vi "Edit Frame.vi"(8 "error in (no error)":errorcluster, 11 "Node Ptr":u64 format="%.0x") -> (0 "error out":errorcluster)   [LabVIEW 2015, in "Diagnostics Addon System Explorer.lvlib"]
uses:
  Diagnostics Addon System Explorer.lvlib
  Types/FG.Action.ctl
  SubVIs/Signal.FG.vi
  Shared/SubVIs/Constants.vi
  <vilib>/NI Veristand/Custom Device API/NI VeriStand - Set Item Property.vi
  <vilib>/NI Veristand/Custom Device API/Set Item Property (U32).vi
  <vilib>/NI Veristand/Custom Device API/Set Item Property (Double).vi
  <vilib>/NI Veristand/Custom Device API/Set Item Property (String).vi
  <vilib>/NI Veristand/Custom Device API/NI VeriStand - Get Item Property.vi
  <vilib>/NI Veristand/Custom Device API/Get Item Property (U32).vi
  <vilib>/NI Veristand/Custom Device API/Get Item Property (Double).vi
  <vilib>/NI Veristand/Custom Device API/Get Item Property (String).vi
  <vilib>/NI Veristand/Custom Device API/NI VeriStand - Get Item Description.vi
  <vilib>/NI Veristand/Custom Device API/NI VeriStand - Get Custom Device Channel Data.vi
  <vilib>/NI Veristand/Custom Device API/Custom Device API.lvlib
  Shared/Diagnostics Addon Shared.lvlib
  <vilib>/NI Veristand/Custom Device Tools/Custom Device Utility Library/Custom Device Utility Library.lvlib
panel:
  in  "Tag":string
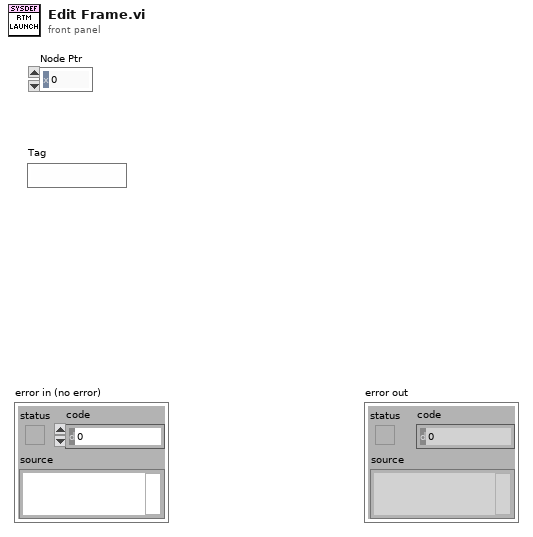
[diagram p1: front panel]
types:
  T1 = typedef "Diagnostics Addon Shared.lvlib/Signal.ctl" = cluster{"Start Bit":u32, "Length":u32, "Scaling Factor":dbl, "Scaling Offset":dbl, "Minimum":dbl, "Maximum":dbl, "Data Type":u32, "Byte Order":u32, "Default Value":dbl, "Name":string, "Units":string, "Description":string}
  T2 = typedef "Custom Device API.lvlib/Custom Device Item Ref.ctl" = u64
  T3 = typedef "Custom Device API.lvlib/Custom Device Item Info.ctl" = cluster{"Name":string, "Is Channel":bool, "GUID":string, "Is Waveform":bool}
  T4 = typedef "Diagnostics Addon System Explorer.lvlib/FG.Action.ctl" = enum16{"Get", "Set"}
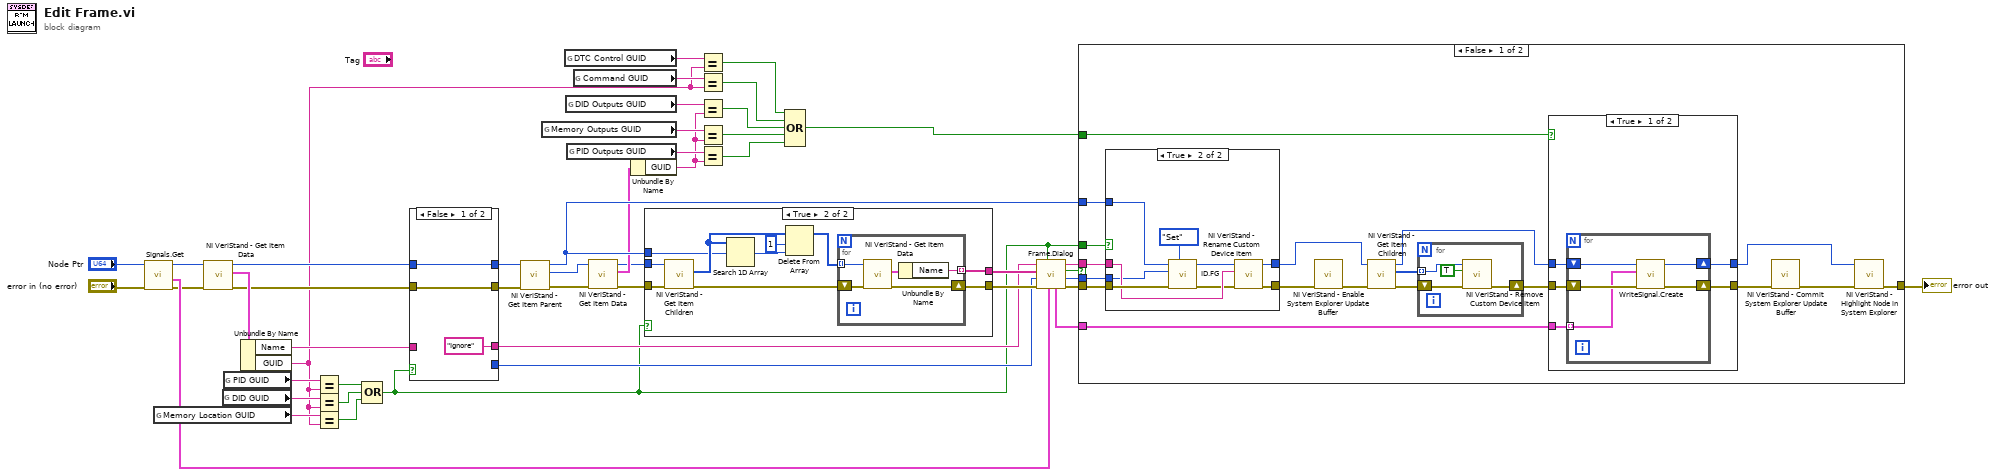
[diagram p0: block diagram]
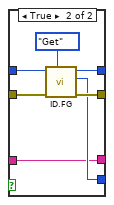
[diagram p3: hidden frame]
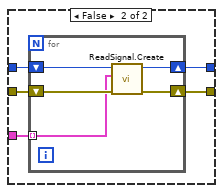
[diagram p5: hidden frame]
diagram:
  n1 = call "Signals.Get.vi"("error in (no error)"="error in (no error)", "Device Item Ref out"="Node Ptr") -> ("error out"=w28:errorcluster, "Parameters"=w30:T1[], "Item Ref out"=w29:T2)  [unwired: 6 in, 1 out]
  n2 = global read "Constants.vi" "Memory Location GUID"() -> (w9:string)
  n3 = call <vilib>:"NI VeriStand - Get Item Data.vi"("error in (no error)"=w28, "Item Ref in"=w29) -> ("error out"=w23:errorcluster, "Item Info"=w26:T3, "Item Ref out"=w24:T2)  [unwired: 6 in, 1 out]
  n4 = global read "Constants.vi" "DID GUID"() -> (w27:string)
  n5 = global read "Constants.vi" "PID GUID"() -> (w25:string)
  n6 = Unbundle By Name(w26) -> ("Name"=w17:string, "GUID"=w4:string)
  n7 = Equal?(x=w25, y=w4) -> (x = y?=w22:bool)
  n8 = Equal?(x=w27, y=w4) -> (x = y?=w21:bool)
  n9 = Equal?(x=w9, y=w4) -> (x = y?=w8:bool)
  n10 = Compound Arithmetic op=OR(w22, w21, w8) -> (w12:bool)
  n11 = case shown="False" w12 {
    tunnel: w24 -> [w49 w52]
    tunnel: w23 -> [w50 w53]
    tunnel: [w50 w56] -> w20
    tunnel: [w49 w55] -> w19
    tunnel: [_ w54] -> w18
    tunnel: ["Ignore" ("Name") w51] -> w16
    tunnel: w17 -> [_ w51]
    frame False {
    }
    frame True {
      n12 = call "ID.FG.vi"("Action"=FG.Action."Get", "error in (no error)"=w53, "Device Item Ref in"=w52) -> ("error out"=w56:errorcluster, "ID"=w54:u32, "Device Item Ref out"=w55:T2)  [unwired: 6 in]
    }
  }
  n13 = call <vilib>:"NI VeriStand - Get Item Parent.vi"("error in (no error)"=w20, "Item Ref in"=w19) -> ("error out"=w38:errorcluster, "Parent Ref"=w37:T2, "Item Ref out"=w42:T2)  [unwired: 6 in, 1 out]
  n14 = global read "Constants.vi" "Memory Outputs GUID"() -> (w10:string)
  n15 = global read "Constants.vi" "DTC Control GUID"() -> (w5:string)
  n16 = global read "Constants.vi" "DID Outputs GUID"() -> (w7:string)
  n17 = global read "Constants.vi" "PID Outputs GUID"() -> (w39:string)
  n18 = global read "Constants.vi" "Command GUID"() -> (w15:string)
  n19 = call <vilib>:"NI VeriStand - Get Item Data.vi"("error in (no error)"=w38, "Item Ref in"=w37) -> ("error out"=w35:errorcluster, "Item Info"=w40:T3, "Item Ref out"=w36:T2)  [unwired: 6 in, 1 out]
  n20 = Unbundle By Name(w40) -> ("GUID"=w6:string)
  n21 = case shown="True" w12 {
    tunnel: [w58 w63] -> w44
    tunnel: [_ w62] -> w43
    tunnel: w42 -> [_ w61]
    tunnel: w36 -> [_ w60]
    tunnel: w35 -> [w58 w59]
    frame False {
    }
    frame True {
      n22 = call <vilib>:"NI VeriStand - Get Item Children.vi"("error in (no error)"=w59, "Item Ref in"=w60) -> ("error out"=w68:errorcluster, "Child Refs"=w67:T2[])  [unwired: 6 in, 2 out]
      n23 = Search 1D Array(1D array=w67, element=w61) -> (index of element=w65:i32)  [unwired: 1 in]
      n24 = Delete From Array(array=w67, length=1, index=w65) -> (array with subset deleted=w66:T2[])  [unwired: 1 out]
      n25 = for {
        tunnel: [w71] -> w62 mode=indexing
        shift-right: [w70] -> w63
        shift-left: w68 -> [w72]
        tunnel: w66 -> [w69] mode=indexing
        n26 = call <vilib>:"NI VeriStand - Get Item Data.vi"("error in (no error)"=w72, "Item Ref in"=w69) -> ("error out"=w70:errorcluster, "Item Info"=w73:T3)  [unwired: 8 out]
        n27 = Unbundle By Name(w73) -> ("Name"=w71:string)
      }
    }
  }
  n28 = Equal?(x=w5, y=w4) -> (x = y?=w1:bool)
  n29 = Equal?(x=w15, y=w4) -> (x = y?=w3:bool)
  n30 = Equal?(x=w7, y=w6) -> (x = y?=w2:bool)
  n31 = Equal?(x=w10, y=w6) -> (x = y?=w11:bool)
  n32 = Equal?(x=w39, y=w6) -> (x = y?=w14:bool)
  n33 = Compound Arithmetic op=OR(w1, w3, w2, w11, w14) -> (w13:bool)
  n34 = call "Frame.Dialog.vi"("Signals"=w30, "Show Name&ID"=w12, "error in (no error)"=w44, "ID"=w18, "Existing PIDs"=w43, "Name"=w16) -> ("error out"=w46:errorcluster, "ID out"=w33:u16, "Cancel PID?"=w45:bool, "Name out"=w47:string, "Signals out"=w34:T1[])  [unwired: 1 in]
  n35 = case shown="False" w45 {
    tunnel: w46 -> [w85 w127]
    tunnel: w47 -> [w83 _]
    tunnel: [w89 w127] -> w41
    tunnel: w42 -> [w86 _]
    tunnel: w13 -> [w87 _]
    tunnel: w34 -> [w84 _]
    tunnel: w33 -> [w82 _]
    tunnel: w12 -> [w79 _]
    frame False {
      n36 = case shown="True" w79 {
        tunnel: w86 -> [w92 w101]
        tunnel: w85 -> [w93 w100]
        tunnel: w83 -> [_ w99]
        tunnel: w82 -> [_ w98]
        tunnel: [w92 w95] -> w76
        tunnel: [w93 w94] -> w78
        frame False {
        }
        frame True {
          n37 = call "ID.FG.vi"("Action"=FG.Action."Set", "error in (no error)"=w100, "ID"=w98, "Device Item Ref in"=w101) -> ("error out"=w97:errorcluster, "Device Item Ref out"=w96:T2)  [unwired: 5 in, 1 out]
          n38 = call <vilib>:"NI VeriStand - Rename Custom Device Item.vi"("error in (no error)"=w97, "New Name"=w99, "Item Ref in"=w96) -> ("error out"=w94:errorcluster, "Item Ref out"=w95:T2)  [unwired: 1 in, 6 out]
        }
      }
      n39 = call <vilib>:"NI VeriStand - Enable System Explorer Update Buffer.vi"("error in (no error)"=w78) -> ("error out"=w77:errorcluster)  [unwired: 10 in]
      n40 = call <vilib>:"NI VeriStand - Get Item Children.vi"("error in (no error)"=w77, "Item Ref in"=w76) -> ("error out"=w90:errorcluster, "Child Refs"=w91:T2[], "Item Ref out"=w80:T2)  [unwired: 6 in, 1 out]
      n41 = for {
        tunnel: w91 -> [w126] mode=indexing
        shift-right: [w123] -> w81
        shift-left: w90 -> [w125]
        n42 = call <vilib>:"NI VeriStand - Remove Custom Device Item.vi"("error in (no error)"=w125, "Force Delete (F)"=TRUE, "Item Ref in"=w126) -> ("error out"=w123:errorcluster)  [unwired: 7 in, 1 out]
      }
      n43 = case shown="True" w87 {
        tunnel: w80 -> [w107 w117]
        tunnel: w84 -> [w106 w116]
        tunnel: [w105 w115] -> w88
        tunnel: w81 -> [w104 w114]
        tunnel: [w103 w113] -> w74
        frame True {
          n44 = for {
            shift-right: [w109] -> w105
            shift-left: w104 -> [w111]
            tunnel: w106 -> [w110] mode=indexing
            shift-right: [w108] -> w103
            shift-left: w107 -> [w112]
            n45 = call "WriteSignal.Create.vi"("error in (no error)"=w111, "Signal Parameters"=w110, "Section Ptr"=w112) -> ("error out"=w109:errorcluster, "Section Ptr out"=w108:T2)  [unwired: 7 in]
          }
        }
        frame False {
          n46 = for {
            shift-right: [w121] -> w115
            shift-left: w114 -> [w122]
            tunnel: w116 -> [w119] mode=indexing
            shift-right: [w118] -> w113
            shift-left: w117 -> [w120]
            n47 = call "ReadSignal.Create.vi"("error in (no error)"=w122, "Signal Parameters"=w119, "Section Ptr"=w120) -> ("error out"=w121:errorcluster, "Section Ptr out"=w118:T2)  [unwired: 7 in]
          }
        }
      }
      n48 = call <vilib>:"NI VeriStand - Commit System Explorer Update Buffer.vi"("error in (no error)"=w88) -> ("error out"=w75:errorcluster)  [unwired: 10 in]
      n49 = call <vilib>:"NI VeriStand - Highlight Node in System Explorer.vi"("error in (no error)"=w75, "Item Ref in"=w74) -> ("error out"=w89:errorcluster)  [unwired: 8 in, 1 out]
    }
    frame True {
    }
  }
  "error out" <- w41
